vi "GLBL_9882_DO_0_3.vi"(10 "9482 DO 0_3":T1, 11 "write_read":bool) -> (2 "9482 DO 0_3 out":T1)   [LabVIEW 2020]
uses:
  controls/DO_0_3.ctl
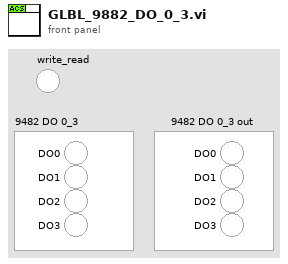
[diagram p1: front panel]
types:
  T1 = typedef "DO_0_3.ctl" = cluster{"DO0":bool, "DO1":bool, "DO2":bool, "DO3":bool}
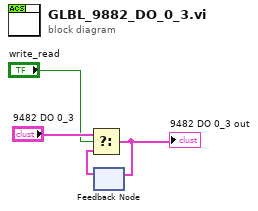
[diagram p0: block diagram]
diagram:
  n1 = feedback #1() -> (w3:T1)  [unwired: 1 in]
  n2 = Select(t="9482 DO 0_3", s="write_read", f=w3) -> (s? t:f=w2:T1)
  "9482 DO 0_3 out" <- w2
  n3 = feedback-in #1(w2) -> ()
